vi "Read error.vi"(8 "error in (no error)":errorcluster, 11 "Error Report in":refnum<class "Error Report.lvclass">) -> (0 "error out":errorcluster, 2 "error":errorcluster, 3 "Error Report out":refnum<class "Error Report.lvclass">)   [LabVIEW 2016, in "Controller API.lvlib" / "Error Result.lvlib" / "Error Report.lvclass"]
uses:
  Error Report.lvclass
  Error Report.lvclass/Error Report.ctl
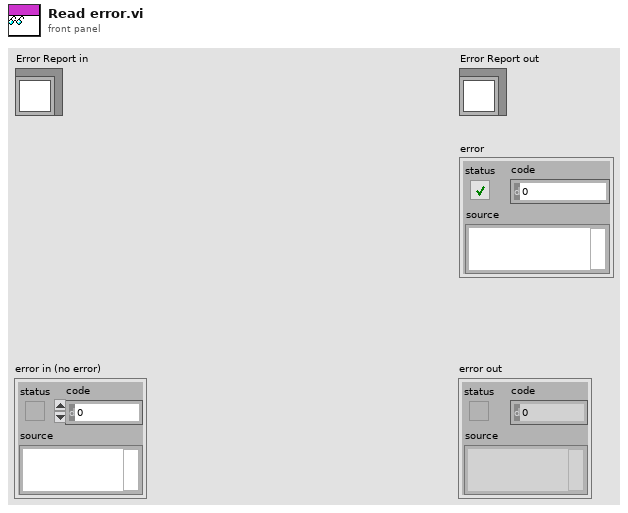
[diagram p1: front panel]
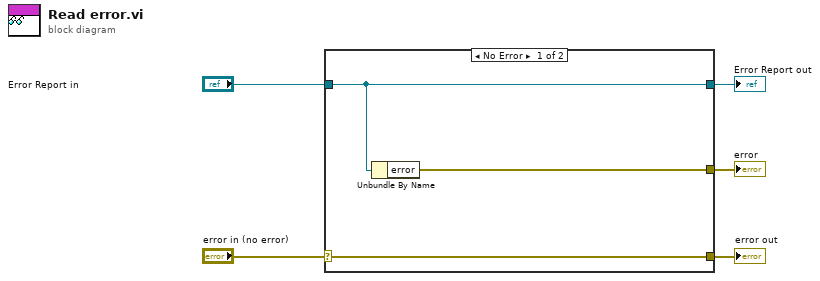
[diagram p0: block diagram]
diagram:
  n1 = case shown="No Error" "error in (no error)" {
    selector: "error in (no error)" -> [w8 w9]
    tunnel: [w8 w9] -> w4
    tunnel: [w7 w10] -> w2
    tunnel: "Error Report in" -> [w7 w10]
    tunnel: [w6 _] -> w1
    frame No Error {
      n2 = Unbundle By Name(w7) -> ("error"=w6:errorcluster)
    }
    frame Error {
    }
  }
  "error out" <- w4
  "Error Report out" <- w2
  "error" <- w1
